vi "Determine Blend Time.vi"(9 "Min R":dbl[](array[numeric]), 11 "WayPoints":cluster{"x":dbl, "y":dbl, "th":dbl}[](array[cluster])) -> (0 "Distance":dbl, 1 "Linear Info":T1(array[cluster]), 2 "Updated Waypoints":cluster{"x":dbl, "y":dbl, "th":dbl}[](array[cluster]), 3 "Blends":T2[](array[typedef]))   [LabVIEW 2025]
uses:
  BlendType.ctl
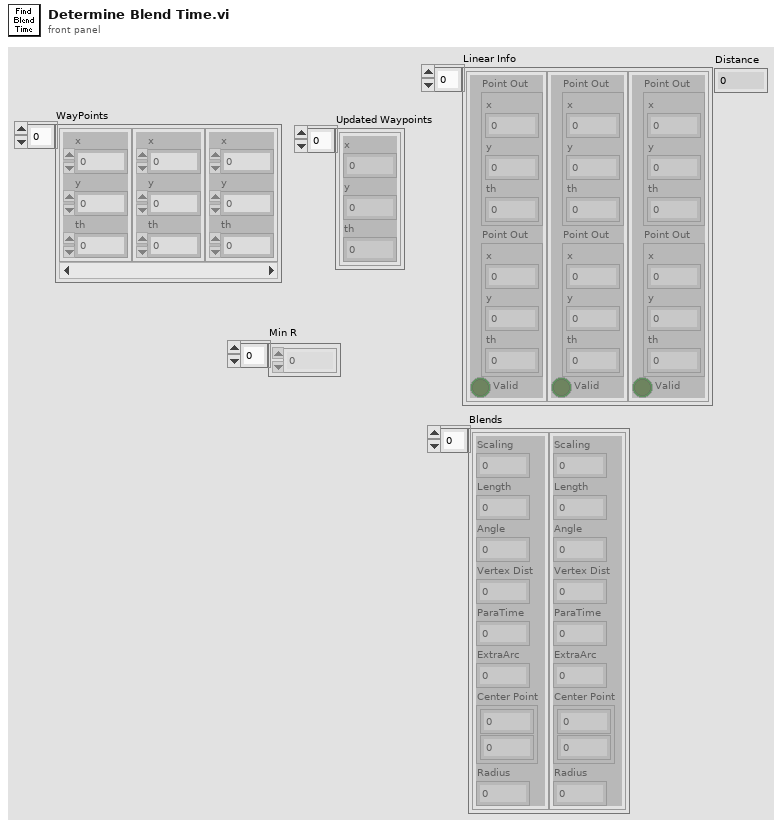
[diagram p1: front panel]
types:
  T1 = cluster{"Point Out":cluster{"x":dbl, "y":dbl, "th":dbl}, "Point Out":cluster{"x":dbl, "y":dbl, "th":dbl}, "Valid":bool}[]
  T2 = typedef "BlendType.ctl" = cluster{"Scaling":dbl, "Length":dbl, "Angle":dbl, "Vertex Dist":dbl, "ParaTime":dbl, "ExtraArc":dbl, "Center Point":cluster{dbl, dbl}, "Radius":dbl}
  T3 = cluster{"Point 1":cluster{"x":dbl, "y":dbl, "th":dbl}, "Point 2":cluster{"x":dbl, "y":dbl, "th":dbl}, bool}[]
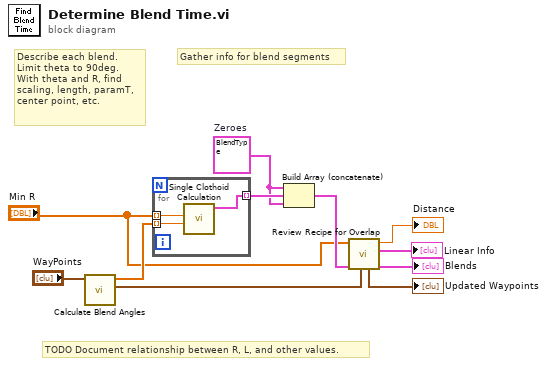
[diagram p0: block diagram]
diagram:
  w7 = T2 {"Scaling"=0.0, "Length"=0.0, "Angle"=0.0, "Vertex Dist"=0.0, "ParaTime"=0.0, "ExtraArc"=0.0, "Center Point"={0.0, 0.0}, "Radius"=0.0}  # Zeroes
  # "Gather info for blend segments"
  # "TODO Document relationship between R, L, and other values."
  # "Describe each blend.\nLimit theta to 90deg.\nWith theta and R, find\nscaling, length, paramT,\ncenter point, etc."
  n1 = call "Calculate Blend Angles.vi"("WayPoints"="WayPoints") -> ("Waypoints out"=w5:cluster{"x":dbl, "y":dbl, "th":dbl}[], "Angles"=w8:dbl[])  [unwired: 9 in]
  n2 = for {
    tunnel: "Min R" -> [w14] mode=indexing
    tunnel: w8 -> [w13] mode=indexing
    tunnel: [w12] -> w9 mode=indexing
    n3 = call "Single Clothoid Calculation.vi"("Angle"=w13, "Min R"=w14) -> ("Zeroes out"=w12:T2)  [unwired: 9 in]
  }
  n4 = Build Array (concatenate)(w7, w9, w7) -> (w2:T2[])
  n5 = call "Review Recipe for Overlap.vi"("Waypoints"=w5, "Blends"=w2, "Min R"="Min R") -> ("Blends out"=→"Blends":T2[], "Linear Info"=→"Linear Info":T3, "Length (f)"=→"Distance":dbl, "Waypoints out"=→"Updated Waypoints":cluster{"x":dbl, "y":dbl, "th":dbl}[])  [unwired: 5 in]
